vi "joystik FGV.vi"() -> ()   [LabVIEW 2019]
uses:
  <vilib>/Utility/inputDevices.llb/joystickAcquire.vi
  <vilib>/Utility/inputDevices.llb/closeJoystick.vi
panel:
  out "error out":errorcluster
  in  "stop":bool
  out "axis info":T1
  out "button info":T2
  out "direction info":T3
  out "Numeric":dbl
  out "Numeric 2":dbl
  out "Numeric 3":dbl
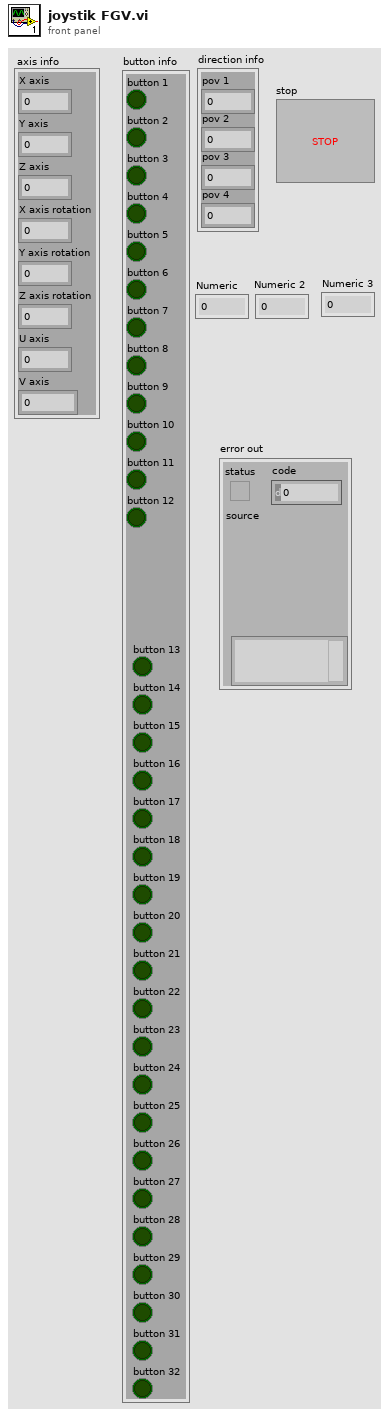
[diagram p1: front panel]
types:
  T1 = cluster{"X axis":i32, "Y axis":i32, "Z axis":i32, "X axis rotation":i32, "Y axis rotation":i32, "Z axis rotation":i32, "U axis":i32, "V axis":i32}
  T2 = cluster{"button 1":bool, "button 2":bool, "button 3":bool, "button 4":bool, "button 5":bool, "button 6":bool, "button 7":bool, "button 8":bool, "button 9":bool, "button 10":bool, "button 11":bool, "button 12":bool, "button 13":bool, "button 14":bool, "button 15":bool, "button 16":bool, "button 17":bool, "button 18":bool, "button 19":bool, "button 20":bool, "button 21":bool, "button 22":bool, "button 23":bool, "button 24":bool, "button 25":bool, "button 26":bool, "button 27":bool, "button 28":bool, "button 29":bool, "button 30":bool, "button 31":bool, "button 32":bool}
  T3 = cluster{"pov 1":i32, "pov 2":i32, "pov 3":i32, "pov 4":i32}
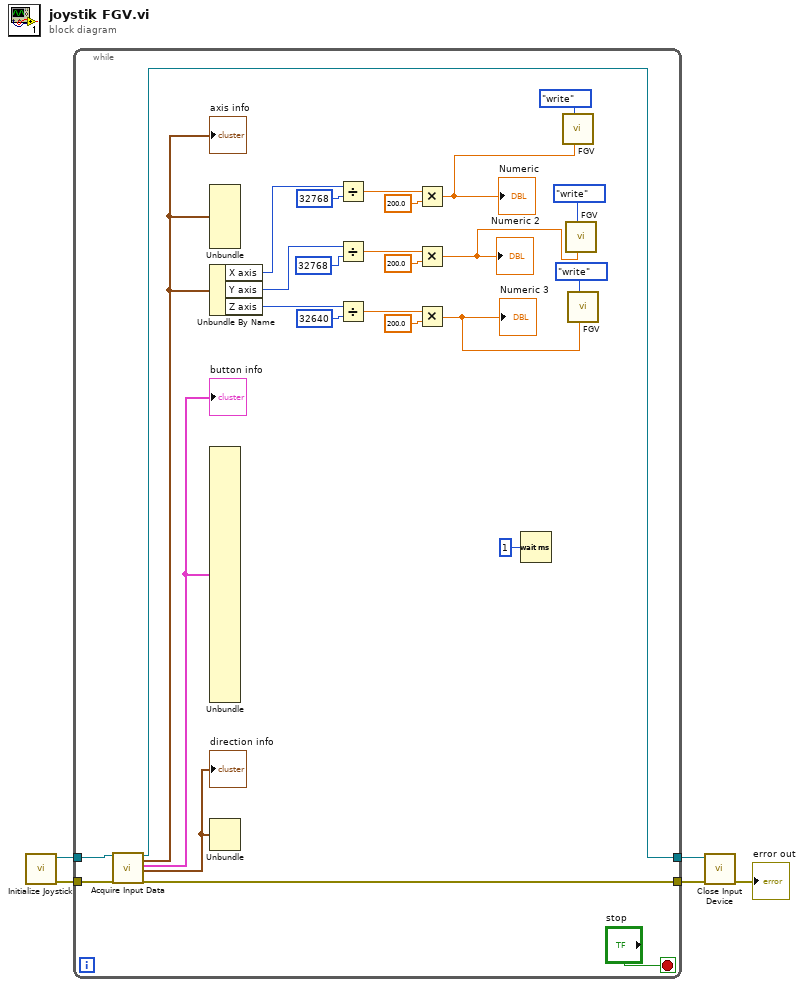
[diagram p0: block diagram]
diagram:
  n1 = call <vilib>:"Initialize Joystick.vi"() -> ("error out"=w2:errorcluster, "device ID"=w5:refnum<k1>)  [unwired: 10 in]
  n2 = while {
    tunnel: [w31] -> w3
    tunnel: [w30] -> w4
    tunnel: w5 -> [w14]
    tunnel: w2 -> [w13]
    stop <- "stop" stop-if-true
    n3 = call-poly <vilib>:"Acquire Input Data.vi"("device ID"=w14, "error in (no error)"=w13) -> ("device ID"=w30:refnum<k1>, "axis info"=w27:T1, "button info"=w29:T2, "direction info"=w28:T3, "error out"=w31:errorcluster)  [unwired: 13 in]
    "axis info" <- w27
    "button info" <- w29
    "direction info" <- w28
    n4 = Unbundle(w27) -> ()  [unwired: 8 out]
    n5 = Unbundle By Name(w27) -> ("X axis"=w26:i32, "Y axis"=w25:i32, "Z axis"=w24:i32)
    n6 = Unbundle(w29) -> ()  [unwired: 32 out]
    n7 = Unbundle(w28) -> ()  [unwired: 4 out]
    n8 = Divide(x=w26, y=32768) -> (x/y=w20:dbl)
    n9 = Divide(x=w25, y=32768) -> (x/y=w18:dbl)
    n10 = Divide(x=w24, y=32640) -> (x/y=w16:dbl)
    n11 = Multiply(x=w20, y=200.0) -> (x*y=w9:dbl)
    "Numeric" <- w9
    n12 = Multiply(x=w18, y=200.0) -> (x*y=w8:dbl)
    "Numeric 2" <- w8
    n13 = Multiply(x=w16, y=200.0) -> (x*y=w6:dbl)
    "Numeric 3" <- w6
    n14 = Wait (ms)(milliseconds to wait=u32 1) -> ()  [unwired: 1 out]
    n15 = call "FGV.vi"("write"=w9, "action"=enum16{"write", "read"}."write") -> ()  [unwired: 9 in, 1 out]
    n16 = call "FGV.vi"("write"=w8, "action"=enum16{"write", "read"}."write") -> ()  [unwired: 9 in, 1 out]
    n17 = call "FGV.vi"("write"=w6, "action"=enum16{"write", "read"}."write") -> ()  [unwired: 9 in, 1 out]
  }
  n18 = call-poly <vilib>:"Close Input Device.vi"("error in (no error)"=w3, "device ID"=w4) -> ("error out"=→"error out":errorcluster)  [unwired: 8 in]
